vi "set step.vi"(8 "error in":errorcluster, 10 "step distance (steps)":dbl format="%#_13g", 11 "actuator in":T1={"Actuator COM"="COM14", "Actuator type"=enum."Scientifica"}) -> (0 "error out":errorcluster, 3 "actuator out":T1={"Actuator COM"="COM14", "Actuator type"=enum."Scientifica"})   [LabVIEW 2015]
uses:
  pipette cleaning/pressure box/cleaning_soft/controls/actuator_type.ctl
  pipette cleaning/pressure box/cleaning_soft/controls/actuator_cluster.ctl
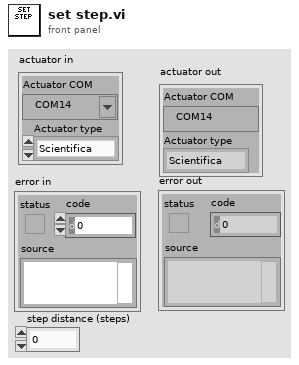
[diagram p1: front panel]
types:
  T1 = typedef "actuator_cluster.ctl" = cluster{"Actuator COM":refnum<visa-resource-name>, "Actuator type":T2}
  T2 = typedef "actuator_type.ctl" = enum16{"Scientifica", "Sutter", "Demo", "Off"}
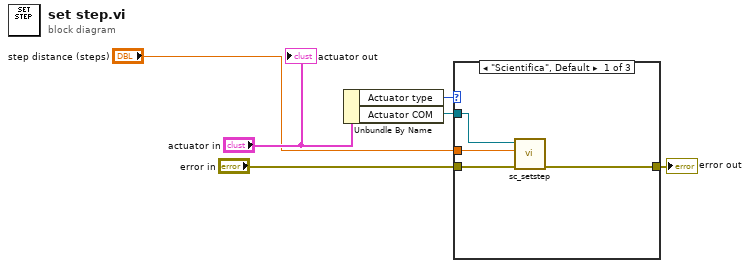
[diagram p0: block diagram]
diagram:
  n1 = Unbundle By Name("actuator in") -> ("Actuator type"=w3:T2, "Actuator COM"=w2:refnum<visa-resource-name>)
  n2 = case shown="\"Scientifica\", Default" w3 {
    tunnel: "error in" -> [w10 w11 w12]
    tunnel: [w9 w11 w12] -> w5
    tunnel: w2 -> [w8 _ _]
    tunnel: "step distance (steps)" -> [w7 _ _]
    frame "Scientifica", Default {
      n3 = call "sc_setstep.vi"("error in"=w10, "step distance (steps)"=w7, "VISA in"=w8) -> ("error out"=w9:errorcluster)  [unwired: 6 in, 2 out]
    }
    frame "Sutter" {
    }
    frame "Demo" {
    }
  }
  "error out" <- w5
  "actuator out" <- "actuator in"
